vi "mod.Test1.vi"(8 "error in":errorcluster, 10 "Data":variant, 11 "Command":string) -> (0 "error out":errorcluster, 3 "Return Data":variant)   [LabVIEW 2014]
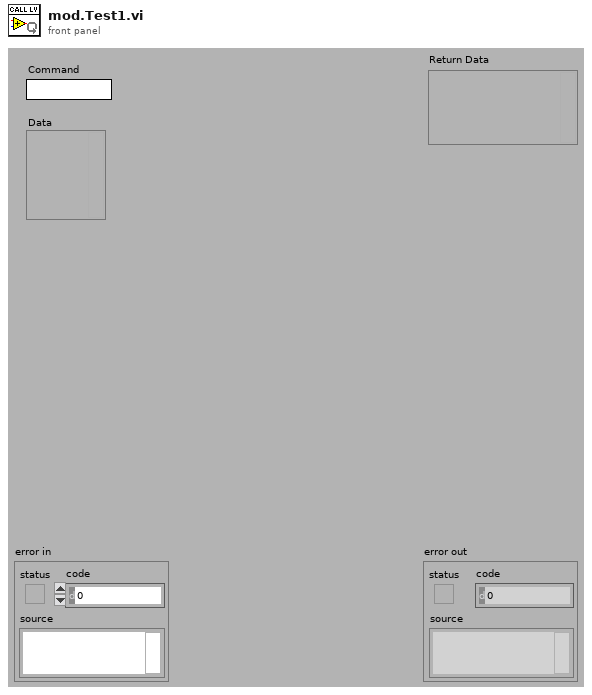
[diagram p1: front panel]
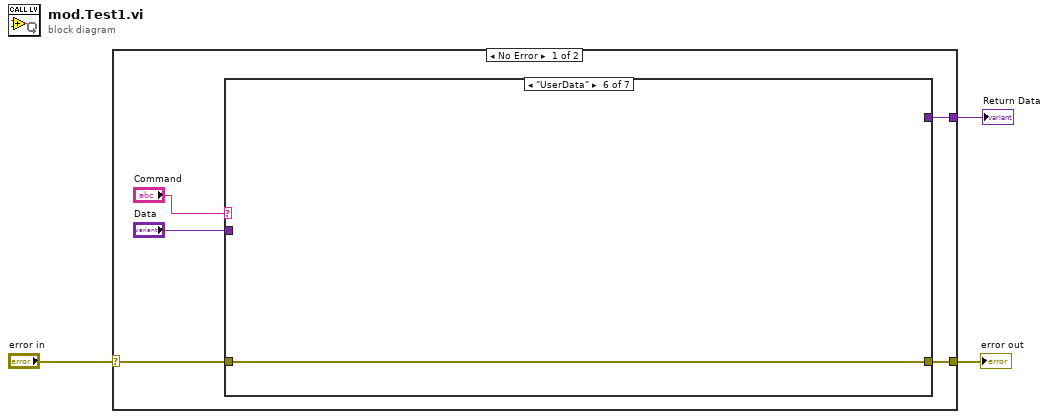
[diagram p0: block diagram]
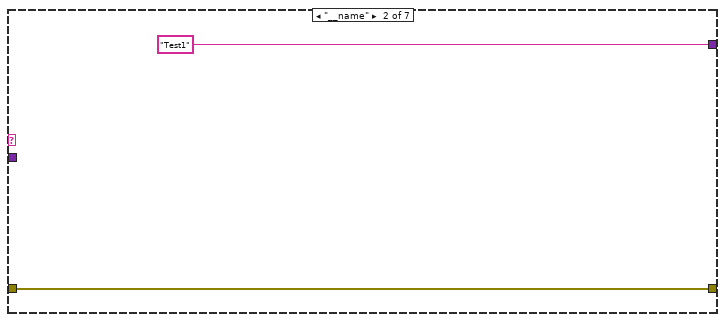
[diagram p3: hidden frame]
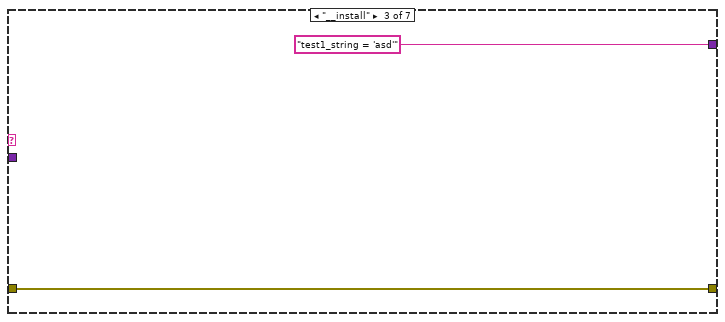
[diagram p4: hidden frame]
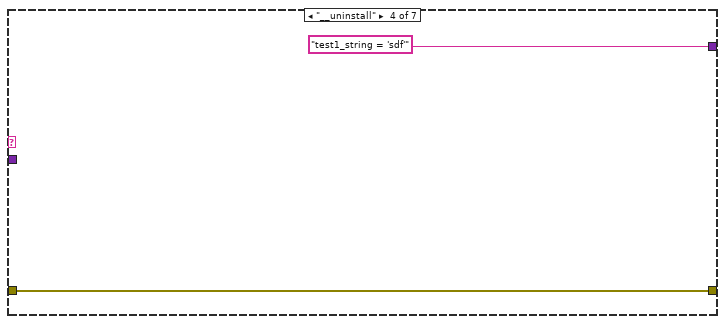
[diagram p5: hidden frame]
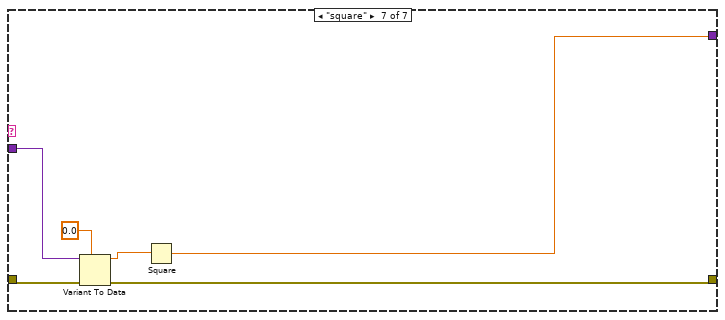
[diagram p7: hidden frame]
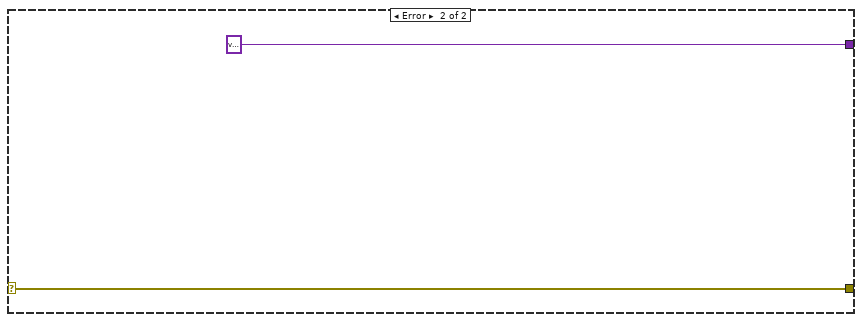
[diagram p8: hidden frame]
diagram:
  n1 = case shown="No Error" "error in" {
    selector: "error in" -> [w8 w27]
    tunnel: [w6 w27] -> w2
    tunnel: [w7 variant ("User Data")] -> w1
    frame No Error {
      n2 = case shown="\"UserData\"" "Command" {
        tunnel: w8 -> [w10 w11 w13 w16 w18 w19 w25]
        tunnel: "Data" -> [w9 _ _ _ w17 _ w24]
        tunnel: [w9 "Test1" "test1_string = 'asd'" "test1_string = 'sdf'" w17 _ w20] -> w7
        tunnel: [w10 w11 w13 w16 w18 w19 w21] -> w6
        frame Default {
        }
        frame "__name" {
        }
        frame "__install" {
        }
        frame "__uninstall" {
        }
        frame "PassThrough" {
        }
        frame "UserData" {
        }
        frame "square" {
          n3 = Variant To Data(error in=w25, type=0.0, Variant=w24) -> (data=w22:dbl, error out=w21:errorcluster)
          n4 = Square(x=w22) -> (x^2=w20:dbl)
        }
      }
    }
    frame Error {
    }
  }
  "Return Data" <- w1
  "error out" <- w2
